vi "compress_exe.vi"(6 "quiet?":bool=TRUE, 8 "error in (no error)":errorcluster, 10 "files_to_add":path, 11 "archive_path in":path) -> (0 "error out":errorcluster, 3 "archive_path out":path)   [LabVIEW 2015, in "lv-bin-7zip.lvlib"]
uses:
  lv-bin-7zip.lvlib
  <userlib>/antonio-alexander/lv-bin/lv-bin/public/api/v1/v1.lvlib
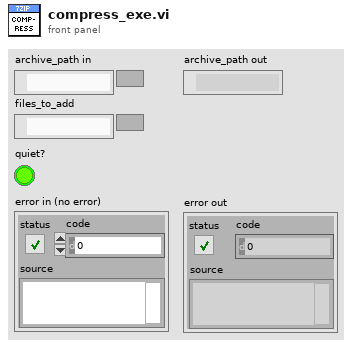
[diagram p1: front panel]
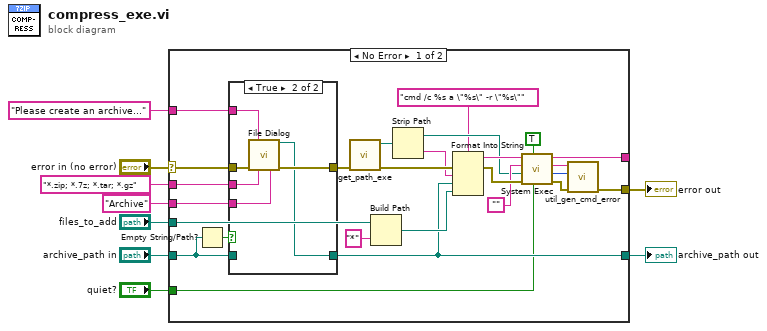
[diagram p0: block diagram]
diagram:
  n1 = case shown="No Error" "error in (no error)" {
    selector: "error in (no error)" -> [w27 w44]
    tunnel: [w15 w44] -> w4
    tunnel: "files_to_add" -> [w11 _]
    tunnel: "archive_path in" -> [w26 _]
    tunnel: "Please create an archive..." ("prompt") -> [w24 _]
    tunnel: [w19 _] -> w5
    tunnel: "*.zip; *.7z; *.tar; *.gz" ("pattern (all files)") -> [w18 _]
    tunnel: "Archive" ("pattern label") -> [w17 _]
    tunnel: "quiet?" -> [w14 _]
    tunnel: [w12 _] -> _
    frame No Error {
      n2 = Empty String/Path?(string/path=w26) -> (empty?=w25:bool)
      n3 = case shown="True" w25 {
        tunnel: w27 -> [w36 w43]
        tunnel: [w36 w42] -> w23
        tunnel: w26 -> [w37 _]
        tunnel: w24 -> [_ w41]
        tunnel: [w37 w40] -> w19
        tunnel: w18 -> [_ w39]
        tunnel: w17 -> [_ w38]
        frame False {
        }
        frame True {
          n4 = call "File Dialog"("prompt"=w41, "error in"=w43, "pattern (all files)"=w39, "pattern label"=w38) -> ("selected path"=w40:path, "error out"=w42:errorcluster)  [unwired: 8 in, 2 out]
        }
      }
      n5 = call "get_path_exe.vi"("error in (no error)"=w23) -> ("error out"=w35:errorcluster, "exe"=w30:path)  [unwired: 9 in]
      n6 = Build Path(base path=w11, name or relative path="*") -> (appended path=w21:path)
      n7 = Strip Path(path=w30) -> (stripped path=w28:path, name=w29:string)
      n8 = Format Into String(format string="cmd /c %s a \"%s\" -r \"%s\"", error in=w35, w29, w19, w21) -> (resulting string=w33:string, error out=w34:errorcluster)  [unwired: 1 in]
      n9 = call <vilib>:"System Exec.vi"("run minimized? (F)"=w14, "wait until completion? (T)"=TRUE, "error in (no error)"=w34, "working directory"=w28, "standard input"="", "command line"=w33) -> ("error out"=w16:errorcluster, "return code"=w10:i32, "standard error"=w13:string, "standard output"=w12:string)  [unwired: 2 in]
      n10 = call <userlib>:"util_gen_cmd_error.vi"("error in (no error)"=w16, "return_code"=w10, "standard_error"=w13) -> ("error out"=w15:errorcluster)  [unwired: 8 in]
    }
    frame Error {
    }
  }
  "error out" <- w4
  "archive_path out" <- w5
